vi "Build Path TimeStamp.vi"(8 "error in":errorcluster, 11 "Report Generator in":refnum<class "Report Generator.lvclass">) -> (0 "error out":errorcluster, 3 "Report Generator out":refnum<class "Report Generator.lvclass">)   [LabVIEW 2018, in "Report Generator.lvlib" / "Report Generator.lvclass"]
uses:
  Report Generator.lvclass
  Report Generator.lvclass/Report Generator.ctl
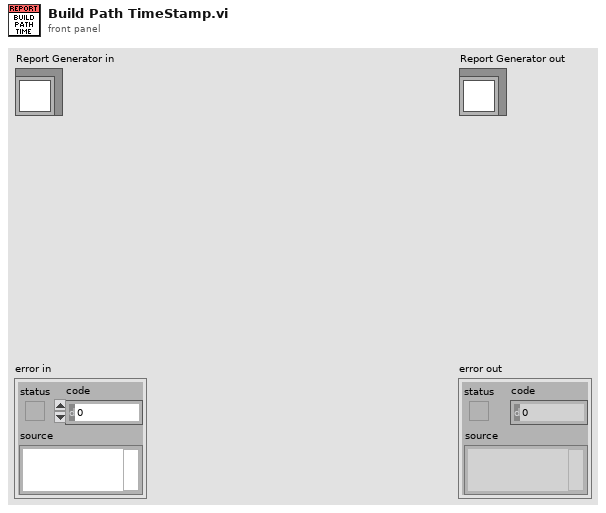
[diagram p1: front panel]
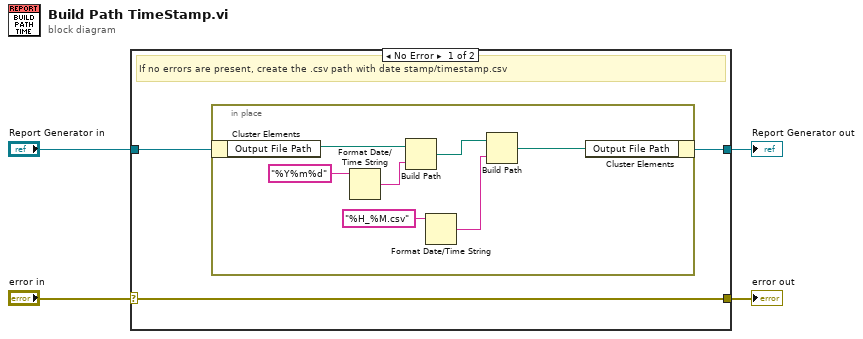
[diagram p0: block diagram]
diagram:
  n1 = case shown="No Error" "error in" {
    selector: "error in" -> [w7 w16]
    tunnel: [w7 w16] -> w3
    tunnel: [w5 w15] -> w1
    tunnel: "Report Generator in" -> [w6 w15]
    frame No Error {
      # "If no errors are present, create the .csv path with date stamp/timestamp.csv"
      n2 = in-place {
        n3 = in-place-cluster #1(w6) -> ("Output File Path"=w14:path)
        n4 = Format Date/Time String(time format string (%c)="%Y%m%d") -> (date/time string=w9:string)  [unwired: 2 in]
        n5 = Build Path(base path=w14, name or relative path=w9) -> (appended path=w13:path)
        n6 = Format Date/Time String(time format string (%c)="%H_%M.csv") -> (date/time string=w8:string)  [unwired: 2 in]
        n7 = Build Path(base path=w13, name or relative path=w8) -> (appended path=w12:path)
        n8 = in-place-cluster #1("Output File Path"=w12) -> (w5:refnum<class "Report Generator.lvclass">)
      }
    }
    frame Error {
    }
  }
  "error out" <- w3
  "Report Generator out" <- w1
